vi "write.vi"(8 "error in (no error)":errorcluster, 10 "String to send":string, 11 "Tektronix RSA5106A in":refnum<class "Tektronix RSA5106A.lvclass">) -> (0 "error out":errorcluster, 3 "Tektronix RSA5106A out":refnum<class "Tektronix RSA5106A.lvclass">)   [LabVIEW 2013, in "Tektronix RSA5106A.lvclass"]
uses:
  Tektronix RSA5106A.lvclass
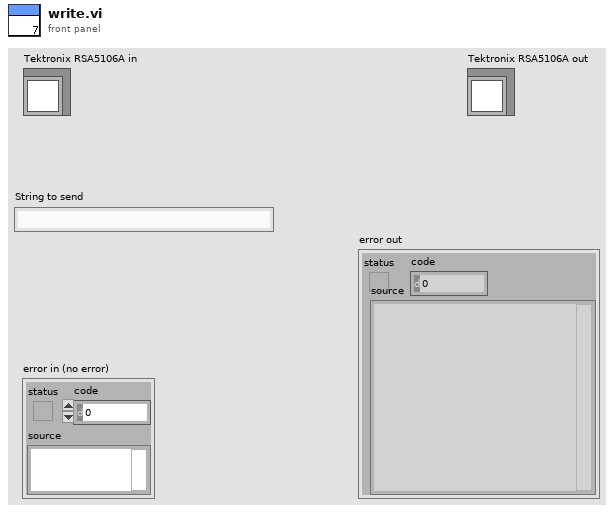
[diagram p1: front panel]
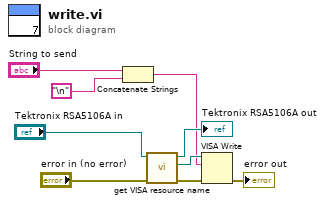
[diagram p0: block diagram]
diagram:
  n1 = Concatenate Strings("String to send", "\n") -> (w2:string)
  n2 = call-dynamic "get VISA resource name.vi"("error in (no error)"="error in (no error)", "DeviceInterface (Eingang)"="Tektronix RSA5106A in") -> ("error out"=w4:errorcluster, "VISA resource name"=w7:refnum<visa-resource-name>, "DeviceInterface (Ausgang)"=→"Tektronix RSA5106A out":refnum<class "Tektronix RSA5106A.lvclass">)  [unwired: 7 in]
  n3 = VISA Write(VISA resource name=w7, write buffer=w2, error in (no error)=w4) -> (error out=→"error out":errorcluster)  [unwired: 2 out]
